vi "Config Format.vi"(11 "Config Path":path) -> (2 "filename without extension":string, 3 "Folder":path, 5 "Format":T1)   [LabVIEW 2020, in "VolatusConfig.lvlib"]
uses:
  VolatusConfig.lvlib
  Config Format.ctl
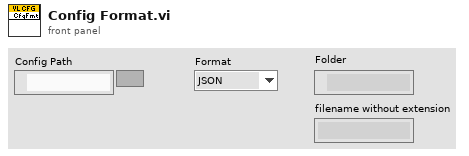
[diagram p1: front panel]
types:
  T1 = typedef "VolatusConfig.lvlib/Config Format.ctl" = enum16{"JSON", "INI", "SQLite"}
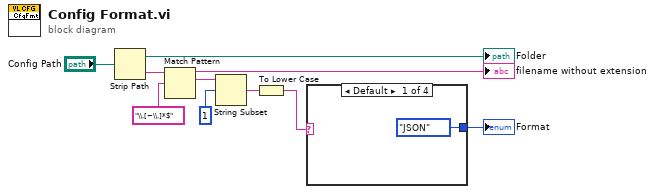
[diagram p0: block diagram]
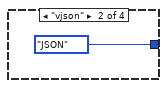
[diagram p2: hidden frame]
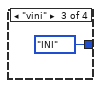
[diagram p3: hidden frame]
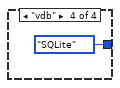
[diagram p4: hidden frame]
diagram:
  n1 = Strip Path(path="Config Path") -> (stripped path=→"Folder":path, name=w2:string)
  n2 = Match Pattern(string=w2, regular expression="\\.[~\\.]*$") -> (before substring=→"filename without extension":string, match substring=w7:string)  [unwired: 3 out]
  n3 = String Subset(string=w7, offset (0)=1) -> (substring=w8:string)  [unwired: 1 out]
  n4 = To Lower Case(string=w8) -> (all lower case string=w5:string)
  n5 = case shown="Default" w5 {
    tunnel: [Config_Format."JSON" ("Config Format") Config_Format."JSON" ("Config Format") Config_Format."INI" ("Config Format") Config_Format."SQLite" ("Config Format")] -> w4
    frame Default {
    }
    frame "vjson" {
    }
    frame "vini" {
    }
    frame "vdb" {
    }
  }
  "Format" <- w4
